vi "SkidpadLapLEDWinker.vi"(8 "inputError":errorcluster, 10 "StateValue":T1, 11 "inputRefOfLED":refnum<vi>[](array[refnum])) -> (0 "outputError":errorcluster)   [LabVIEW 2020]
uses:
  Control/SkidpadState.ctl
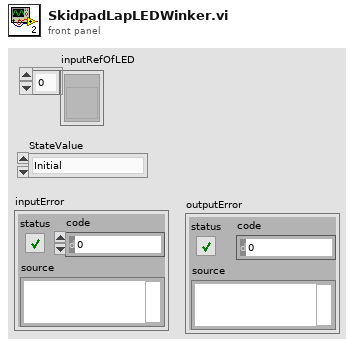
[diagram p1: front panel]
types:
  T1 = typedef "SkidpadState.ctl" = enum16{"Initial", "InputInfomation", "Ready", "1lap", "2lap", "3lap", "4lap", "FinshRunning", "LogRecord", "HardwareRelease", "WaittingforNext", "ProgramStop"}
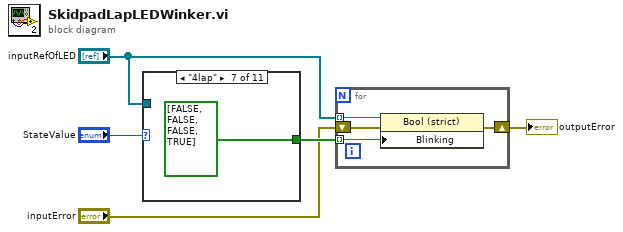
[diagram p0: block diagram]
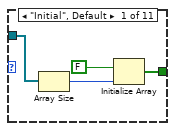
[diagram p2: hidden frame]
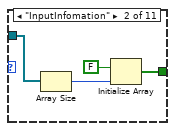
[diagram p3: hidden frame]
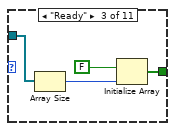
[diagram p4: hidden frame]
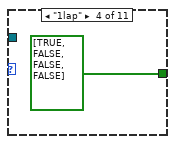
[diagram p5: hidden frame]
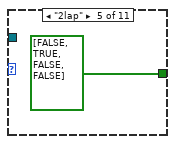
[diagram p6: hidden frame]
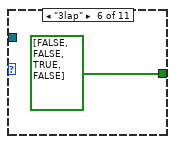
[diagram p7: hidden frame]
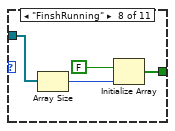
[diagram p8: hidden frame]
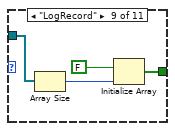
[diagram p9: hidden frame]
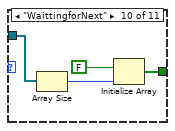
[diagram p10: hidden frame]
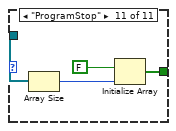
[diagram p11: hidden frame]
diagram:
  n1 = case shown="\"4lap\"" "StateValue" {
    tunnel: "inputRefOfLED" -> [w8 w12 w16 _ _ _ _ w24 w28 w32 w36]
    tunnel: [w5 w9 w13 bool[] [TRUE, FALSE, FALSE, FALSE] bool[] [FALSE, TRUE, FALSE, FALSE] bool[] [FALSE, FALSE, TRUE, FALSE] bool[] [FALSE, FALSE, FALSE, TRUE] w21 w25 w29 w33] -> w4
    frame "Initial", Default {
      n2 = Array Size(array=w8) -> (size(s)=w7:i32)
      n3 = Initialize Array "Initialize Array"(FALSE, w7) -> (w5:bool[])
    }
    frame "InputInfomation" {
      n4 = Array Size(array=w12) -> (size(s)=w11:i32)
      n5 = Initialize Array "Initialize Array"(FALSE, w11) -> (w9:bool[])
    }
    frame "Ready" {
      n6 = Array Size(array=w16) -> (size(s)=w15:i32)
      n7 = Initialize Array "Initialize Array"(FALSE, w15) -> (w13:bool[])
    }
    frame "1lap" {
    }
    frame "2lap" {
    }
    frame "3lap" {
    }
    frame "4lap" {
    }
    frame "FinshRunning" {
      n8 = Array Size(array=w24) -> (size(s)=w23:i32)
      n9 = Initialize Array "Initialize Array"(FALSE, w23) -> (w21:bool[])
    }
    frame "LogRecord" {
      n10 = Array Size(array=w28) -> (size(s)=w27:i32)
      n11 = Initialize Array "Initialize Array"(FALSE, w27) -> (w25:bool[])
    }
    frame "WaittingforNext" {
      n12 = Array Size(array=w32) -> (size(s)=w31:i32)
      n13 = Initialize Array "Initialize Array"(FALSE, w31) -> (w29:bool[])
    }
    frame "ProgramStop" {
      n14 = Array Size(array=w36) -> (size(s)=w35:i32)
      n15 = Initialize Array "Initialize Array"(FALSE, w35) -> (w33:bool[])
    }
  }
  n16 = for {
    shift-right: [w39] -> _
    shift-left: _ -> [w40]
    tunnel: w4 -> [w38] mode=indexing
    tunnel: "inputRefOfLED" -> [w37] mode=indexing
    n17 = property class="Bool (strict)"(reference=w37, error in=w40, "Blinking"=w38) -> (error out=w39:errorcluster)  [unwired: 1 out]
  }
  "outputError" <- "inputError"
